vi "五参数标样核查.vi"(11 "启动参数":T1={"测量模式"="标样核查", "数据类型"="N", "输出参数"={"水温"=FALSE, "pH"=FALSE, "DO"=FALSE, "浊度"=FALSE, "电导率"=FALSE}}) -> ()   [LabVIEW 2016, in "斯坦道原位多参数.lvlib"]
panel:
  out "枚举":T2(ring)
  out "状态":string
  out "数值":i32
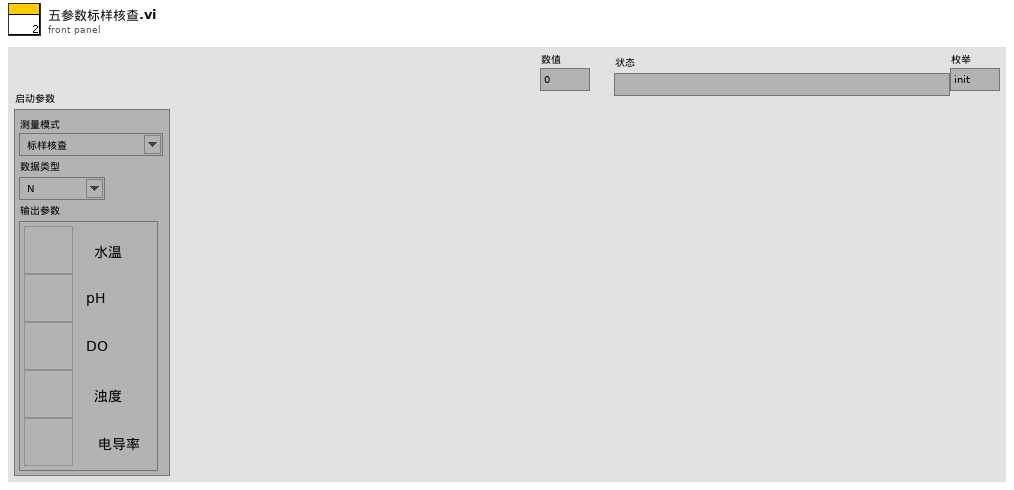
[diagram p1: front panel]
types:
  T1 = typedef "斯坦道原位多参数.lvlib/标样核查启动自定义输入参数.ctl" = cluster{"测量模式":string, "数据类型":string, "输出参数":cluster{"水温":bool, "pH":bool, "DO":bool, "浊度":bool, "电导率":bool}}
  T2 = enum16{"init", "开机", "启动测量", "读取测量值", "存储数据", "关闭测量", "关机", "结束"}
  T3 = cluster{"时间标识":timestamp, "设备":string, "日志信息":string, "流程参数":string}
  T4 = cluster{"系统时间":timestamp, "工作状态":u16, "测量模式":u16, "告警代码":enum16{"无告警", "缺试剂告警", "缺水样告警", "缺蒸馏水告警", "缺标液告警", "仪表漏液告警", "标定异常告警", "超量程告警", "加热异常", "低试剂预警", "超上限告警", "超下限告警", "仪表内部其他异常", "滴定异常告警", "电极异常告警", "量程切换告警", "参数设置告警", "PH电极电位异常", "电导率电极异常", "浊度光度异常", "溶解氧电极异常", "溶解氧光强异常", "温度异常告警", "PH异常告警", "溶解氧异常告警", "电导率异常告警", "浊度异常告警", "叶绿素异常告警", "藻密度异常告警", "蓝绿藻异常告警", "ORP异常告警", "氨氮异常告警", "清洁刷异常告警", "SD卡异常告警", "蓝牙异常告警", "Wifi异常告警", "流程异常告警"}, "故障代码":enum16{"无故障", "电机故障", "温度故障", "通讯故障", "滴定故障"}, "日志代码":u16, "软件版本":string}
  T5 = cluster{"水温标准液标准浓度":dbl, "酸碱度标准液标准浓度":dbl, "溶解氧标准液标准浓度":dbl, "电导率标准液标准浓度":dbl, "浊度标准液标准浓度":dbl}
  T6 = cluster{"因子编码":string, "单位":string, "标样参考值":sgl, "水样数据时间":timestamp, "水样实测值":sgl, "水样数据标识":string, "K":sgl, "B":sgl, "T":sgl, "H":sgl, "水深":sgl, "探头温度":sgl, "信号值":sgl}
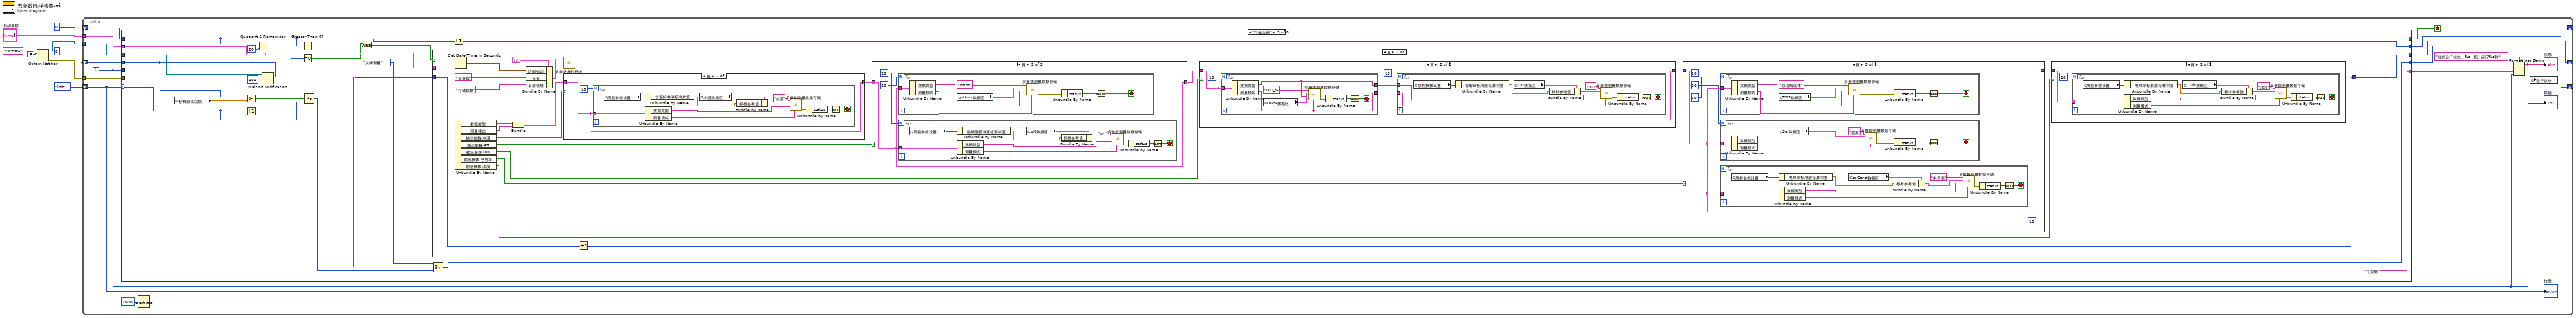
[diagram p0: block diagram]
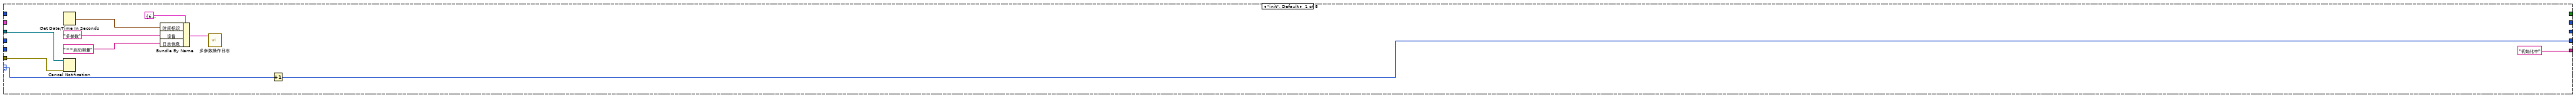
[diagram p2: hidden frame]
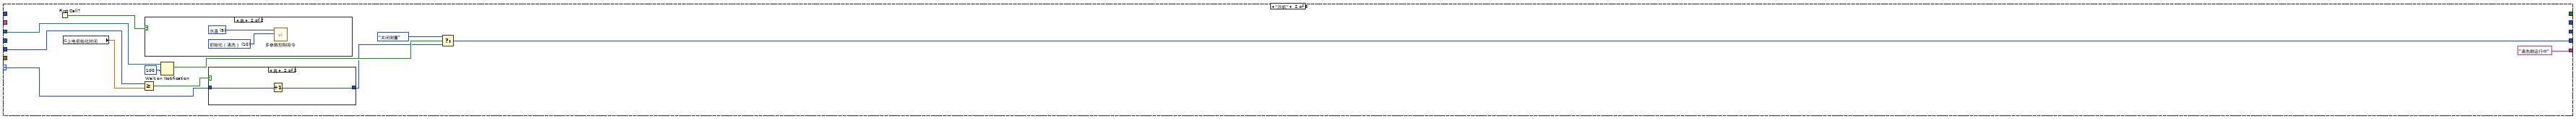
[diagram p3: hidden frame]
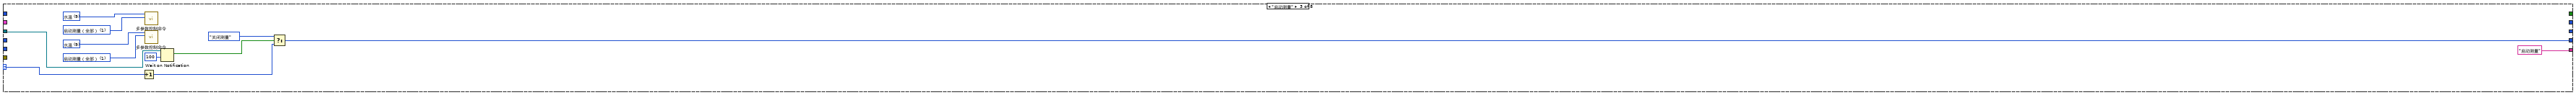
[diagram p6: hidden frame]
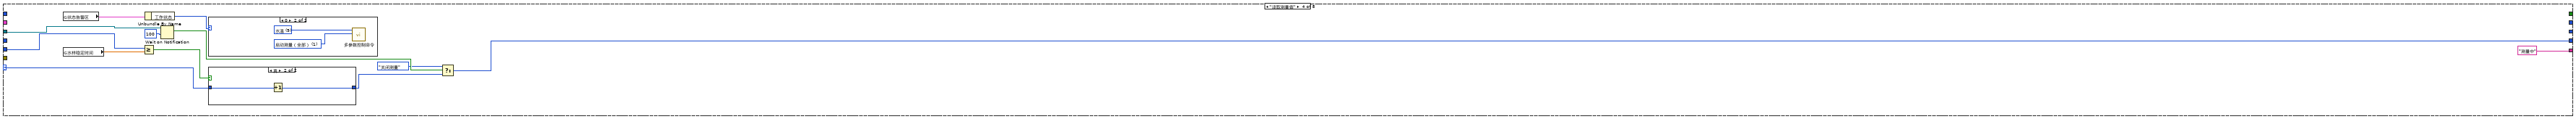
[diagram p7: hidden frame]
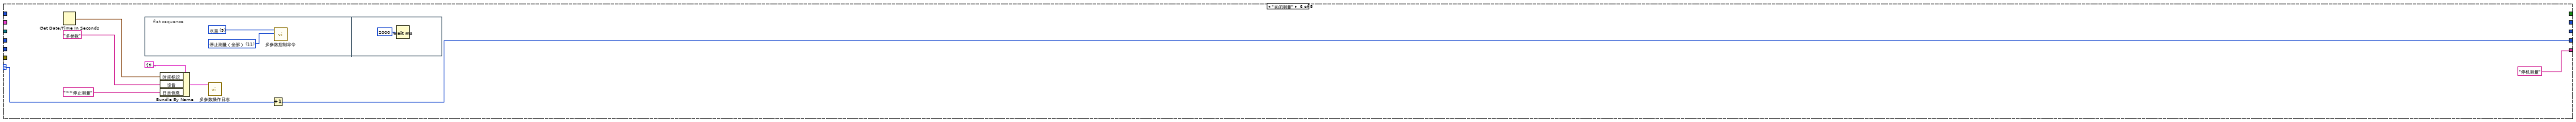
[diagram p16: hidden frame]
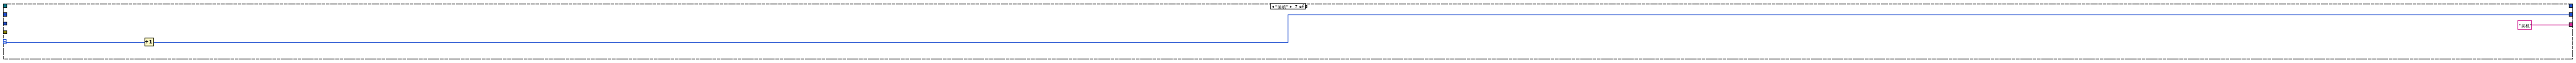
[diagram p17: hidden frame]
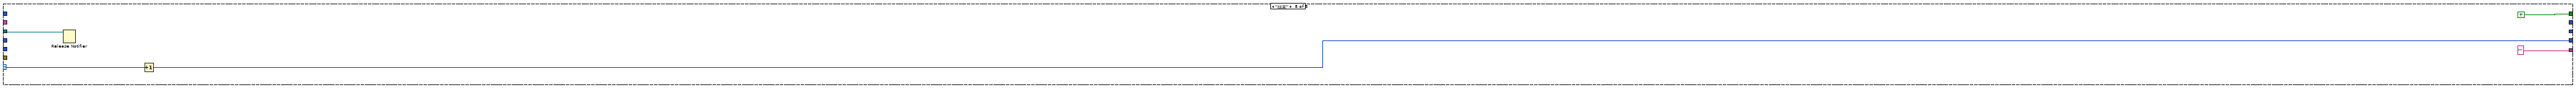
[diagram p18: hidden frame]
diagram:
  n1 = Obtain Notifier(name (unnamed)="MPFlow" ("名称（未命名）"), notification data type=FALSE) -> (notifier out=w5:refnum<notifier>, error out=w4:errorcluster)  [unwired: 2 in, 1 out]
  n2 = while {
    shift-right: [w19] -> _
    shift-left: T2."init" ("枚举") -> [w23]
    tunnel: w5 -> [w21]
    tunnel: w4 -> [w20]
    tunnel: "启动参数" -> [w13]
    shift-right: [w11] -> _
    shift-left: u32 0 ("等待时间（毫秒）") -> [w12]
    shift-right: [w9] -> _
    shift-left: u32 0 ("等待时间（毫秒）") -> [w10]
    i -> [w15]
    stop <- w22 stop-if-true
    n3 = case shown="\"存储数据\"" w23 {
      selector: w23 -> [w31 w45 w62 w75 w82 w236 w242 w246]
      tunnel: [_ _ _ _ _ _ _ TRUE] -> w22
      tunnel: w21 -> [w33 w41 w61 w72 w91 _ _ w243]
      tunnel: w20 -> [w32 _ _ _ _ _ _ _]
      tunnel: [w30 w39 w58 w70 w87 w235 w241 w245] -> w19
      tunnel: w15 -> [_ w44 _ w66 _ _ _ _]
      tunnel: ["初始化中" ("状态") "清洗刷运行中" ("状态") "启动测量" ("状态") "测量中" ("状态") "存数据" ("状态") "停机测量" ("状态") "关机" ("状态") "" ("状态")] -> w16
      tunnel: w13 -> [_ _ _ _ w100 _ _ _]
      tunnel: w12 -> [_ _ _ _ w94 _ _ _]
      tunnel: [_ _ _ _ w95 _ _ _] -> w11
      tunnel: w10 -> [_ _ _ _ w84 _ _ _]
      tunnel: [_ _ _ _ w86 _ _ _] -> w9
      frame "init", Default {
        n4 = Get Date/Time In Seconds() -> (seconds since 1Jan1904=w27:timestamp)
        n5 = Cancel Notification(0:w33, 3:w32) -> ()  [unwired: 3 out]
        n6 = Bundle By Name(cluster=T3 {"时间标识"=timestamp(0 s since 1904-01-01), "设备"="", "日志信息"="", "流程参数"=""} ("data in"), "时间标识"=w27, "设备"="多参数", "日志信息"="<<启动测量") -> (w26:T3)
        n7 = call "多参数操作日志.vi"("data"=w26) -> ()  [unwired: 10 in, 1 out]
        n8 = Increment(x=w31) -> (x+1=w30:T2)
      }
      frame "开机" {
        n9 = First Call?() -> (First Call?: T/F=w35:bool)
        n10 = global read "多参数断电保存全局变量.vi" "上电初始化时间"() -> (w34:dbl)
        n11 = Greater Or Equal?(x=w44, y=w34) -> (x >= y?=w43:bool)
        n12 = case shown="真" w35 {
          frame False {
          }
          frame True {
            w47 = u16 10 items=["启动测量（全部）"=1, "初始化（清洗）"=10, "停止测量（全部）"=11, "校时"=13, "启动测量（单个传感器）"=19, "停止测量（单个传感器）"=20] ("控制命令")
            w46 = u16 9 items=["氨氮"=3, "水温"=9, "pH值"=10, "溶解氧"=11, "电导率"=12, "浊度"=13, "叶绿素a"=14, "藻密度"=15, "蓝绿藻"=16, "氧化还原电位"=17, "溶解氧%"=18, "盐度"=19] ("站号")
            n13 = call "多参数控制命令.vi"("控制命令"=w47, "站号"=w46) -> ()  [unwired: 9 in, 1 out]
          }
        }
        n14 = Wait on Notification(notifier=w41, timeout in ms (-1)=100 ("超时毫秒(-1)")) -> (notification=w42:bool)  [unwired: 2 in, 3 out]
        n15 = case shown="真" w43 {
          tunnel: w45 -> [w48 w50]
          tunnel: [w48 w49] -> w40
          frame False {
          }
          frame True {
            n16 = Increment(x=w50) -> (x+1=w49:T2)
          }
        }
        n17 = Select(t=T2."关闭测量" ("枚举"), s=w42, f=w40) -> (s? t:f=w39:T2)
      }
      frame "启动测量" {
        w52 = u16 1 items=["启动测量（全部）"=1, "初始化（清洗）"=10, "停止测量（全部）"=11, "校时"=13, "启动测量（单个传感器）"=19, "停止测量（单个传感器）"=20] ("控制命令")
        w51 = u16 9 items=["氨氮"=3, "水温"=9, "pH值"=10, "溶解氧"=11, "电导率"=12, "浊度"=13, "叶绿素a"=14, "藻密度"=15, "蓝绿藻"=16, "氧化还原电位"=17, "溶解氧%"=18, "盐度"=19] ("站号")
        w53 = u16 1 items=["启动测量（全部）"=1, "初始化（清洗）"=10, "停止测量（全部）"=11, "校时"=13, "启动测量（单个传感器）"=19, "停止测量（单个传感器）"=20] ("控制命令")
        w54 = u16 9 items=["氨氮"=3, "水温"=9, "pH值"=10, "溶解氧"=11, "电导率"=12, "浊度"=13, "叶绿素a"=14, "藻密度"=15, "蓝绿藻"=16, "氧化还原电位"=17, "溶解氧%"=18, "盐度"=19] ("站号")
        n18 = Increment(x=w62) -> (x+1=w59:T2)
        n19 = call "多参数控制命令.vi"("控制命令"=w52, "站号"=w51) -> ()  [unwired: 9 in, 1 out]
        n20 = call "多参数控制命令.vi"("控制命令"=w53, "站号"=w54) -> ()  [unwired: 9 in, 1 out]
        n21 = Wait on Notification(notifier=w61, timeout in ms (-1)=100 ("超时毫秒(-1)")) -> (notification=w60:bool)  [unwired: 2 in, 3 out]
        n22 = Select(t=T2."关闭测量" ("枚举"), s=w60, f=w59) -> (s? t:f=w58:T2)
      }
      frame "读取测量值" {
        n23 = global read "多参数全局变量.vi" "状态告警区"() -> (w65:T4)
        n24 = global read "多参数断电保存全局变量.vi" "水样稳定时间"() -> (w63:dbl)
        n25 = Greater Or Equal?(x=w66, y=w63) -> (x >= y?=w74:bool)
        n26 = Unbundle By Name(w65) -> ("工作状态"=w64:u16)
        n27 = Wait on Notification(notifier=w72, timeout in ms (-1)=100 ("超时毫秒(-1)")) -> (notification=w73:bool)  [unwired: 2 in, 3 out]
        n28 = case shown="0" w64 {
          frame Default {
          }
          frame 0 {
            w76 = u16 1 items=["启动测量（全部）"=1, "初始化（清洗）"=10, "停止测量（全部）"=11, "校时"=13, "启动测量（单个传感器）"=19, "停止测量（单个传感器）"=20] ("控制命令")
            w77 = u16 9 items=["氨氮"=3, "水温"=9, "pH值"=10, "溶解氧"=11, "电导率"=12, "浊度"=13, "叶绿素a"=14, "藻密度"=15, "蓝绿藻"=16, "氧化还原电位"=17, "溶解氧%"=18, "盐度"=19] ("站号")
            n29 = call "多参数控制命令.vi"("控制命令"=w76, "站号"=w77) -> ()  [unwired: 9 in, 1 out]
          }
        }
        n30 = case shown="真" w74 {
          tunnel: w75 -> [w78 w80]
          tunnel: [w78 w79] -> w71
          frame False {
          }
          frame True {
            n31 = Increment(x=w80) -> (x+1=w79:T2)
          }
        }
        n32 = Select(t=T2."关闭测量" ("枚举"), s=w73, f=w71) -> (s? t:f=w70:T2)
      }
      frame "存储数据" {
        n33 = global read "多参数断电保存全局变量.vi" "标样测试组数"() -> (w81:dbl)
        n34 = Greater Or Equal?(x=w84, y=w81) -> (x >= y?=w85:bool)
        n35 = Increment(x=w82) -> (x+1=w83:T2)
        n36 = Quotient & Remainder(x=w94, y=u32 60) -> (x-y*floor(x/y)=w98:u32)  [unwired: 1 out]
        n37 = Wait on Notification(notifier=w91, timeout in ms (-1)=100 ("超时毫秒(-1)")) -> (notification=w90:bool)  [unwired: 2 in, 3 out]
        n38 = Greater Than 0?(x=w94) -> (x > 0?=w93:bool)
        n39 = Equal To 0?(x=w98) -> (x = 0?=w97:bool)
        n40 = Select(t=w83, s=w85, f=w82) -> (s? t:f=w89:T2)
        n41 = Compound Arithmetic op=AND ("复合运算")(w97, w93) -> (w96:bool)
        n42 = Select(t=T2."关闭测量", s=w90, f=w89) -> (s? t:f=w87:T2)
        n43 = case shown="真" w96 {
          tunnel: w100 -> [_ w122]
          tunnel: w84 -> [w102 w104]
          tunnel: [w102 w103] -> w86
          frame False {
          }
          frame True {
            n44 = Get Date/Time In Seconds() -> (seconds since 1Jan1904=w113:timestamp)
            n45 = Unbundle By Name(w122) -> ("数据类型"=w121:string, "测量模式"=w120:string, "输出参数.水温"=w109:bool, "输出参数.pH"=w108:bool, "输出参数.DO"=w107:bool, "输出参数.电导率"=w106:bool, "输出参数.浊度"=w105:bool)
            n46 = Bundle("数据类型"=w121, "测量模式"=w120) -> (w119:cluster{"数据类型":string, "测量模式":string})  [unwired: 1 in]
            n47 = Bundle By Name(cluster=T3 {"时间标识"=timestamp(0 s since 1904-01-01), "设备"="", "日志信息"="", "流程参数"=""} ("data in"), "时间标识"=w113, "设备"="多参数", "日志信息"="存储数据") -> (w112:T3)
            n48 = call "多参数操作日志.vi"("data"=w112) -> ()  [unwired: 10 in, 1 out]
            n49 = case shown="真" w109 {
              tunnel: w119 -> [w215 w217]
              tunnel: [w215 w217] -> w118
              frame False {
              }
              frame True {
                n50 = for {
                  N: 10 -> [_]
                  tunnel: w217 -> [w228]
                  stop <- w222 stop-if-true
                  n51 = global read "多参数断电保存全局变量.vi" "质控参数设置"() -> (w226:T5)
                  n52 = Unbundle By Name(w226) -> ("水温标准液标准浓度"=w225:dbl)
                  n53 = Unbundle By Name(w228) -> ("数据类型"=w219:string, "测量模式"=w218:string)
                  n54 = global read "多参数全局变量.vi" "水温数据区"() -> (w227:T6)
                  n55 = Bundle By Name(cluster=w227, "标样参考值"=w225) -> (w221:T6)
                  n56 = call "多参数测量数据存储.vi"("测量模式"=w218, "数据类型"=w219, "数据区"=w221, "table输入"="水温") -> ("error out"=w224:errorcluster)  [unwired: 7 in]
                  n57 = Unbundle By Name(w224) -> ("status"=w223:bool)
                  n58 = Not(x=w223) -> (.not. x?=w222:bool)
                }
              }
            }
            n59 = Increment(x=w104) -> (x+1=w103:u32)
            n60 = case shown="真" w108 {
              tunnel: w118 -> [w192 w195]
              tunnel: [w192 w195] -> w116
              frame False {
              }
              frame True {
                n61 = for {
                  N: 10 -> [_]
                  tunnel: w195 -> [w203]
                  stop <- w200 stop-if-true
                  n62 = Unbundle By Name(w203) -> ("数据类型"=w197:string, "测量模式"=w196:string)
                  n63 = global read "多参数全局变量.vi" "pHmv数据区"() -> (w198:T6)
                  n64 = call "多参数测量数据存储.vi"("测量模式"=w196, "数据类型"=w197, "数据区"=w198, "table输入"="pHmv") -> ("error out"=w202:errorcluster)  [unwired: 7 in]
                  n65 = Unbundle By Name(w202) -> ("status"=w201:bool)
                  n66 = Not(x=w201) -> (.not. x?=w200:bool)
                }
                n67 = for {
                  N: 10 -> [_]
                  tunnel: w195 -> [w214]
                  stop <- w208 stop-if-true
                  n68 = global read "多参数断电保存全局变量.vi" "质控参数设置"() -> (w213:T5)
                  n69 = Unbundle By Name(w213) -> ("酸碱度标准液标准浓度"=w212:dbl)
                  n70 = Unbundle By Name(w214) -> ("数据类型"=w205:string, "测量模式"=w204:string)
                  n71 = global read "多参数全局变量.vi" "pH数据区"() -> (w211:T6)
                  n72 = Bundle By Name(cluster=w211, "标样参考值"=w212) -> (w206:T6)
                  n73 = call "多参数测量数据存储.vi"("测量模式"=w204, "数据类型"=w205, "数据区"=w206, "table输入"="pH") -> ("error out"=w210:errorcluster)  [unwired: 7 in]
                  n74 = Unbundle By Name(w210) -> ("status"=w209:bool)
                  n75 = Not(x=w209) -> (.not. x?=w208:bool)
                }
              }
            }
            n76 = case shown="真" w107 {
              tunnel: [w168 w173] -> w117
              tunnel: w116 -> [w168 w173]
              frame False {
              }
              frame True {
                n77 = for {
                  N: 10 -> [_]
                  tunnel: w173 -> [w191]
                  tunnel: [w185] -> w172
                  tunnel: [w184] -> w171
                  stop <- w188 stop-if-true
                  n78 = Unbundle By Name(w191) -> ("数据类型"=w184:string, "测量模式"=w185:string)
                  n79 = global read "多参数全局变量.vi" "DO%数据区"() -> (w186:T6)
                  n80 = call "多参数测量数据存储.vi"("测量模式"=w185, "数据类型"=w184, "数据区"=w186, "table输入"="DO_%") -> ("error out"=w190:errorcluster)  [unwired: 7 in]
                  n81 = Unbundle By Name(w190) -> ("status"=w189:bool)
                  n82 = Not(x=w189) -> (.not. x?=w188:bool)
                }
                n83 = for {
                  N: 10 -> [_]
                  tunnel: w172 -> [w174]
                  tunnel: w171 -> [w177]
                  stop <- w178 stop-if-true
                  n84 = global read "多参数断电保存全局变量.vi" "质控参数设置"() -> (w183:T5)
                  n85 = Unbundle By Name(w183) -> ("溶解氧标准液标准浓度"=w182:dbl)
                  n86 = global read "多参数全局变量.vi" "DO数据区"() -> (w181:T6)
                  n87 = Bundle By Name(cluster=w181, "标样参考值"=w182) -> (w175:T6)
                  n88 = call "多参数测量数据存储.vi"("测量模式"=w174, "数据类型"=w177, "数据区"=w175, "table输入"="DO") -> ("error out"=w180:errorcluster)  [unwired: 7 in]
                  n89 = Unbundle By Name(w180) -> ("status"=w179:bool)
                  n90 = Not(x=w179) -> (.not. x?=w178:bool)
                }
              }
            }
            n91 = case shown="真" w106 {
              tunnel: w117 -> [w136 w140]
              tunnel: [w136 w140] -> w115
              frame False {
              }
              frame True {
                (unwired) 10
                n92 = for {
                  N: 10 -> [_]
                  tunnel: w140 -> [w148]
                  stop <- w145 stop-if-true
                  n93 = Unbundle By Name(w148) -> ("数据类型"=w142:string, "测量模式"=w141:string)
                  n94 = global read "多参数全局变量.vi" "TDS数据区"() -> (w143:T6)
                  n95 = call "多参数测量数据存储.vi"("测量模式"=w141, "数据类型"=w142, "数据区"=w143, "table输入"="总溶解固体") -> ("error out"=w147:errorcluster)  [unwired: 7 in]
                  n96 = Unbundle By Name(w147) -> ("status"=w146:bool)
                  n97 = Not(x=w146) -> (.not. x?=w145:bool)
                }
                n98 = for {
                  N: 10 -> [_]
                  tunnel: w140 -> [w167]
                  stop <- w164 stop-if-true
                  n99 = Unbundle By Name(w167) -> ("数据类型"=w161:string, "测量模式"=w160:string)
                  n100 = global read "多参数全局变量.vi" "Sal数据区"() -> (w162:T6)
                  n101 = call "多参数测量数据存储.vi"("测量模式"=w160, "数据类型"=w161, "数据区"=w162, "table输入"="盐度") -> ("error out"=w166:errorcluster)  [unwired: 7 in]
                  n102 = Unbundle By Name(w166) -> ("status"=w165:bool)
                  n103 = Not(x=w165) -> (.not. x?=w164:bool)
                }
                n104 = for {
                  N: 10 -> [_]
                  tunnel: w140 -> [w159]
                  stop <- w153 stop-if-true
                  n105 = global read "多参数断电保存全局变量.vi" "质控参数设置"() -> (w158:T5)
                  n106 = Unbundle By Name(w158) -> ("电导率标准液标准浓度"=w157:dbl)
                  n107 = Unbundle By Name(w159) -> ("数据类型"=w150:string, "测量模式"=w149:string)
                  n108 = global read "多参数全局变量.vi" "spCond数据区"() -> (w156:T6)
                  n109 = Bundle By Name(cluster=w156, "标样参考值"=w157) -> (w151:T6)
                  n110 = call "多参数测量数据存储.vi"("测量模式"=w149, "数据类型"=w150, "数据区"=w151, "table输入"="电导率") -> ("error out"=w155:errorcluster)  [unwired: 7 in]
                  n111 = Unbundle By Name(w155) -> ("status"=w154:bool)
                  n112 = Not(x=w154) -> (.not. x?=w153:bool)
                }
              }
            }
            n113 = case shown="真" w105 {
              tunnel: w115 -> [_ w124]
              frame False {
              }
              frame True {
                n114 = for {
                  N: 10 -> [_]
                  tunnel: w124 -> [w135]
                  stop <- w129 stop-if-true
                  n115 = global read "多参数断电保存全局变量.vi" "质控参数设置"() -> (w134:T5)
                  n116 = Unbundle By Name(w134) -> ("电导率标准液标准浓度"=w133:dbl)
                  n117 = Unbundle By Name(w135) -> ("数据类型"=w126:string, "测量模式"=w125:string)
                  n118 = global read "多参数全局变量.vi" "Turb数据区"() -> (w132:T6)
                  n119 = Bundle By Name(cluster=w132, "标样参考值"=w133) -> (w127:T6)
                  n120 = call "多参数测量数据存储.vi"("测量模式"=w125, "数据类型"=w126, "数据区"=w127, "table输入"="浊度") -> ("error out"=w131:errorcluster)  [unwired: 7 in]
                  n121 = Unbundle By Name(w131) -> ("status"=w130:bool)
                  n122 = Not(x=w130) -> (.not. x?=w129:bool)
                }
              }
            }
          }
        }
        n123 = Increment(x=w94) -> (x+1=w95:u32)
      }
      frame "关闭测量" {
        n124 = Get Date/Time In Seconds() -> (seconds since 1Jan1904=w232:timestamp)
        n125 = flat-sequence {
          frame #0 {
            w237 = u16 11 items=["启动测量（全部）"=1, "初始化（清洗）"=10, "停止测量（全部）"=11, "校时"=13, "启动测量（单个传感器）"=19, "停止测量（单个传感器）"=20] ("控制命令")
            w238 = u16 9 items=["氨氮"=3, "水温"=9, "pH值"=10, "溶解氧"=11, "电导率"=12, "浊度"=13, "叶绿素a"=14, "藻密度"=15, "蓝绿藻"=16, "氧化还原电位"=17, "溶解氧%"=18, "盐度"=19] ("站号")
            n126 = call "多参数控制命令.vi"("控制命令"=w237, "站号"=w238) -> ()  [unwired: 9 in, 1 out]
          }
          frame #1 {
            n127 = Wait (ms)(milliseconds to wait=u32 2000 ("等待时间（毫秒）")) -> ()  [unwired: 1 out]
          }
        }
        n128 = Bundle By Name(cluster=T3 {"时间标识"=timestamp(0 s since 1904-01-01), "设备"="", "日志信息"="", "流程参数"=""} ("data in"), "时间标识"=w232, "设备"="多参数", "日志信息"=">>停止测量") -> (w231:T3)
        n129 = call "多参数操作日志.vi"("data"=w231) -> ()  [unwired: 10 in, 1 out]
        n130 = Increment(x=w236) -> (x+1=w235:T2)
      }
      frame "关机" {
        n131 = Increment(x=w242) -> (x+1=w241:T2)
      }
      frame "结束" {
        n132 = Release Notifier(notifier=w243) -> ()  [unwired: 2 in, 3 out]
        n133 = Increment(x=w246) -> (x+1=w245:T2)
      }
    }
    n134 = Wait (ms)(milliseconds to wait=u32 1000 ("等待时间（毫秒）")) -> ()  [unwired: 1 out]
    n135 = Format Into String(format string="当前运行状态：%s  累计运行%d秒" ("格式字符串"), w16, w15) -> (resulting string=w14:string)  [unwired: 2 in, 1 out]
    "状态" <- w14
    n136 = global write "多参数全局变量.vi" "运行状态"(w14) -> ()
    "数值" <- w15
    "枚举" <- w23
  }
